vi "Configure Sequencer Marker Delays.vi"(5 "Marker 4 (0.0)":dbl format="%^.3e", 6 "Marker 3 (0.0)":dbl format="%^.3e", 7 "Marker 2 (0.0)":dbl format="%^.3e", 8 "error in (no error)":errorcluster, 9 "Restart Marker (0.0)":dbl format="%^.3e", 10 "Instance (1)":i32=1, 11 "VISA resource name":refnum<visa-resource-name>) -> (0 "error out":errorcluster, 3 "VISA resource name out":refnum<visa-resource-name>)   [LabVIEW 2015, in "Rohde&Schwarz CMXP GPRF.lvlib"]
doc: "Defines delay times for the ARB output trigger events relative to the marker events.\n\nAttribute:\nRSCMXPGPRF_ATTR_SEQUENCER_MARKER_DELAYS\n\nRemote-control command:\nSOURce:GPRF:GEN<i>:SEQuencer:MARKer:DELays"
uses:
  <instrlib>/Rohde&Schwarz CMXP GPRF/Rohde&Schwarz CMXP GPRF.lvlib
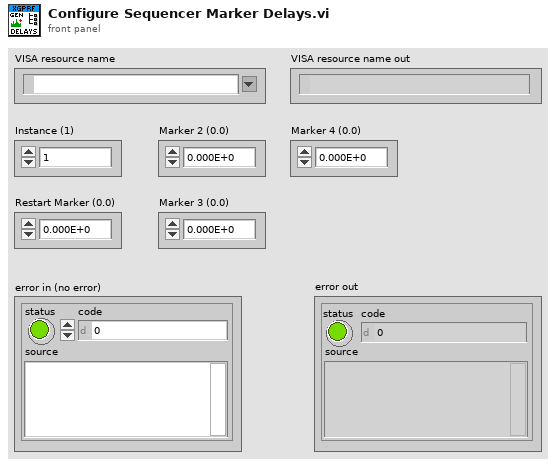
[diagram p1: front panel]
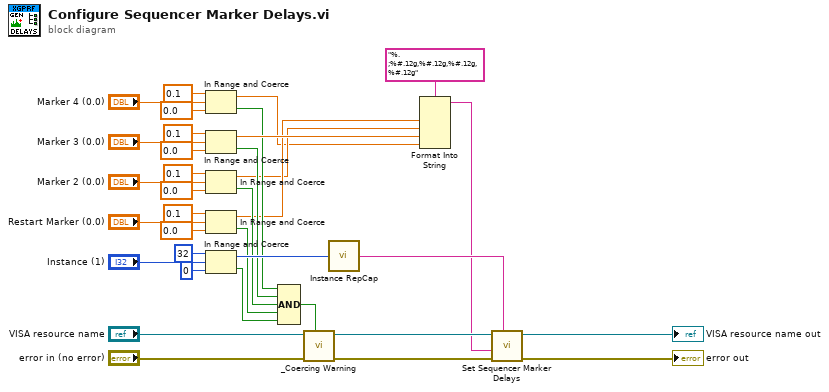
[diagram p0: block diagram]
diagram:
  n1 = In Range and Coerce(upper limit=0.1, x="Marker 4 (0.0)", lower limit=0.0) -> (coerced(x)=w2:dbl, In Range?=w5:bool)
  n2 = In Range and Coerce(upper limit=0.1, x="Marker 3 (0.0)", lower limit=0.0) -> (coerced(x)=w11:dbl, In Range?=w6:bool)
  n3 = In Range and Coerce(upper limit=0.1, x="Marker 2 (0.0)", lower limit=0.0) -> (coerced(x)=w3:dbl, In Range?=w7:bool)
  n4 = In Range and Coerce(upper limit=0.1, x="Restart Marker (0.0)", lower limit=0.0) -> (coerced(x)=w4:dbl, In Range?=w8:bool)
  n5 = In Range and Coerce(upper limit=32, x="Instance (1)", lower limit=0) -> (coerced(x)=w12:i32, In Range?=w9:bool)
  n6 = Compound Arithmetic op=AND(w5, w6, w7, w8, w9) -> (w18:bool)
  n7 = call <instrlib>:"_Coercing Warning.vi"("In Range?"=w18, "error in (no error)"="error in (no error)", "VISA resource name"="VISA resource name") -> ("error out"=w16:errorcluster, "VISA resource name out"=w15:refnum<visa-resource-name>)  [unwired: 7 in]
  n8 = call <instrlib>:"Instance RepCap.vi"("Instance in"=w12) -> ("Instance out"=w10:string)
  n9 = Format Into String(format string="%.;%#.12g,%#.12g,%#.12g,%#.12g", w4, w3, w11, w2) -> (resulting string=w1:string)  [unwired: 2 in, 1 out]
  n10 = call "Set Sequencer Marker Delays"("Repeated Capabilities"=w10, "error in (no error)"=w16, "Sequencer Marker Delays ()"=w1, "instrument handle"=w15) -> ("error out"=→"error out":errorcluster, "instrument handle out"=→"VISA resource name out":refnum<visa-resource-name>)  [unwired: 6 in]
